vi "Clear Image.vi"(8 "error in (no error)":errorcluster, 11 "Reference Control in":refnum<class "Reference Control.lvclass">) -> (0 "error out":errorcluster, 3 "Reference Control out":refnum<class "Reference Control.lvclass">)   [LabVIEW 2016, in "Reference Control.lvclass"]
uses:
  Reference Control.lvclass
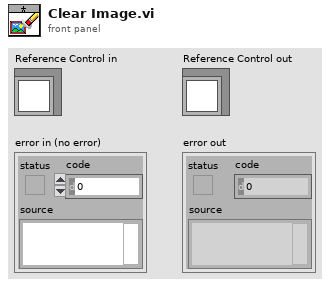
[diagram p1: front panel]
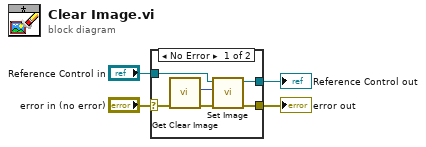
[diagram p0: block diagram]
diagram:
  n1 = case shown="No Error" "error in (no error)" {
    selector: "error in (no error)" -> [w8 w12]
    tunnel: [w7 w12] -> w3
    tunnel: [w5 w11] -> w1
    tunnel: "Reference Control in" -> [w6 w11]
    frame No Error {
      n2 = call "Get Clear Image.vi"("error in (no error)"=w8) -> ("error out"=w9:errorcluster, "Picture"=w10:picture)  [unwired: 9 in]
      n3 = call "Set Image.vi"("error in (no error)"=w9, "Picture"=w10, "Reference Control in"=w6) -> ("error out"=w7:errorcluster, "Reference Control out"=w5:refnum<class "Reference Control.lvclass">)  [unwired: 7 in]
    }
    frame Error {
    }
  }
  "error out" <- w3
  "Reference Control out" <- w1
